vi "CRYSet ViewProperty XY  Front Panel.vi"(11 "Vi Ref":refnum<vi>) -> ()   [LabVIEW 2013]
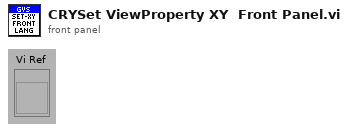
[diagram p1: front panel]
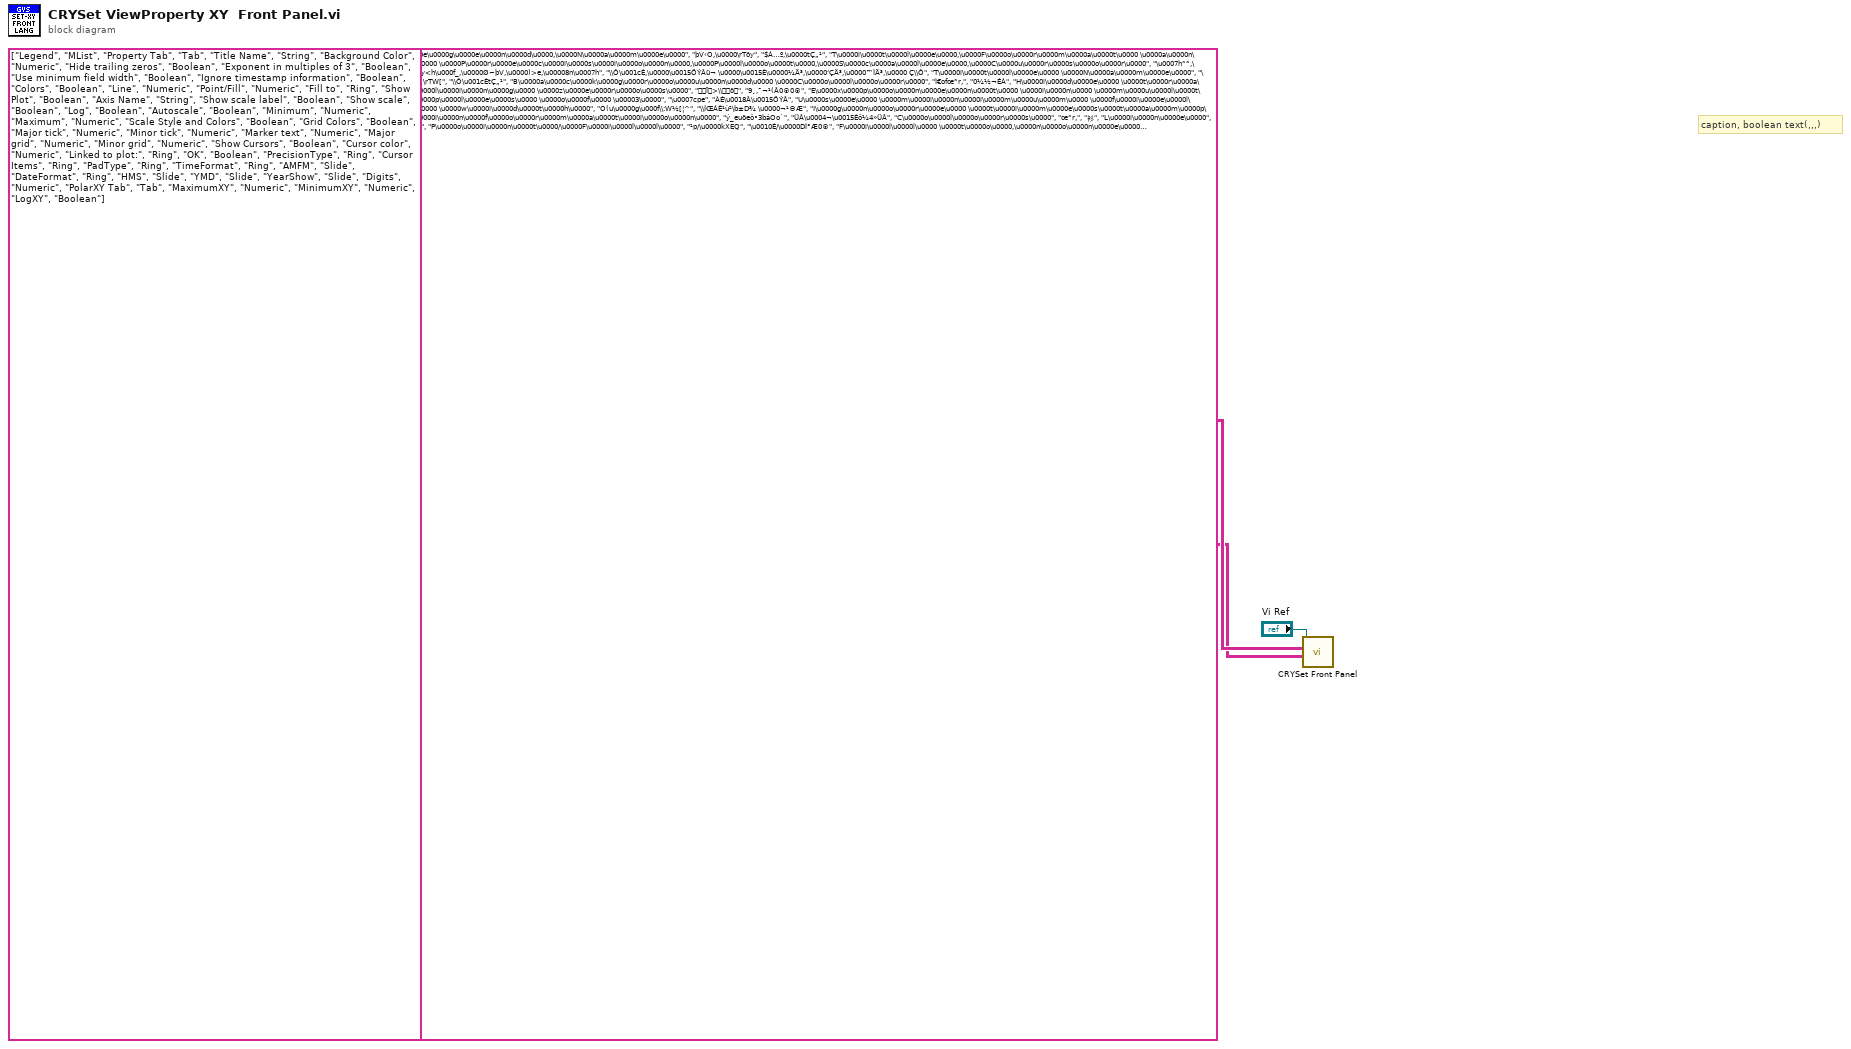
[diagram p0: block diagram]
diagram:
  # "Caption, Tab Page, Multilist Header, Button 4"
  # "Control Type"
  # "Control Name and Tab"
  # "caption, boolean text(,,,)"
  # "Caption/Boolean Text"
  n1 = call "CRYSet Front Panel.vi"("Caption(Boolean Text)"=string[][] [["L\u0000e\u0000g\u0000e\u0000n\u0000d\u0000,\u0000N\u0000a\u0000m\u0000e\u0000", "þV‹O,\u0000\rTðy", "$Á…º,\u0000tÇ„¹"], ["T\u0000i\u0000t\u0000l\u0000e\u0000,\u0000F\u0000o\u0000r\u0000m\u0000a\u0000t\u0000 \u0000a\u0000n\u0000d\u0000 \u0000P\u0000r\u0000e\u0000c\u0000i\u0000s\u0000i\u0000o\u0000n\u0000,\u0000P\u0000l\u0000o\u0000t\u0000,\u0000S\u0000c\u0000a\u0000l\u0000e\u0000,\u0000C\u0000u\u0000r\u0000s\u0000o\u0000r\u0000", "\u0007h˜˜,\u0000>f:y<h\u000f_,\u0000Ø~þV,\u0000)>e,\u00008n\u0007h", "\\Ô\u001cÈ,\u0000\u0015ÖÝÂü¬ \u0000\u0015È\u0000¼Ä³,\u0000‘ÇÄ³,\u0000™ÌÄ³,\u0000 Ç\\Ô"], ["T\u0000i\u0000t\u0000l\u0000e\u0000 \u0000N\u0000a\u0000m\u0000e\u0000", "\u0007h˜˜\rTW[", "\\Ô\u001cÈtÇ„¹"], ["B\u0000a\u0000c\u0000k\u0000g\u0000r\u0000o\u0000u\u0000n\u0000d\u0000 \u0000C\u0000o\u0000l\u0000o\u0000r\u0000", "Ì€ofœ˜r‚", "0¼½¬ÉÀ"], ["H\u0000i\u0000d\u0000e\u0000 \u0000t\u0000r\u0000a\u0000i\u0000l\u0000i\u0000n\u0000g\u0000 \u0000z\u0000e\u0000r\u0000o\u0000s\u0000", "Ï>\\ö", "9¸,¯¬¹(Â0®0®"], ["E\u0000x\u0000p\u0000o\u0000n\u0000e\u0000n\u0000t\u0000 \u0000i\u0000n\u0000 \u0000m\u0000u\u0000l\u0000t\u0000i\u0000p\u0000l\u0000e\u0000s\u0000 \u0000o\u0000f\u0000 \u00003\u0000", "\u0007cpe", "ÀÉ\u0018Â\u0015ÖÝÂ"], ["U\u0000s\u0000e\u0000 \u0000m\u0000i\u0000n\u0000i\u0000m\u0000u\u0000m\u0000 \u0000f\u0000i\u0000e\u0000l\u0000d\u0000 \u0000w\u0000i\u0000d\u0000t\u0000h\u0000", "O(u\u0000g\u000f\\:W½[¦^", "\\ÍŒÁÈ¹ù²\b±D¾ \u0000¬¹©Æ"], ["I\u0000g\u0000n\u0000o\u0000r\u0000e\u0000 \u0000t\u0000i\u0000m\u0000e\u0000s\u0000t\u0000a\u0000m\u0000p\u0000 \u0000i\u0000n\u0000f\u0000o\u0000r\u0000m\u0000a\u0000t\u0000i\u0000o\u0000n\u0000", "ý_euöeô•3báOo`", "ÜÂ\u0004¬\u0015Èô¼4»ÜÂ"], ["C\u0000o\u0000l\u0000o\u0000r\u0000s\u0000", "œ˜r‚", "衫"], ["L\u0000i\u0000n\u0000e\u0000", "¿~", " Á"], ["P\u0000o\u0000i\u0000n\u0000t\u0000/\u0000F\u0000i\u0000l\u0000l\u0000", "¹p/\u0000kXEQ", "\u0010È/\u0000DÌ°Æ0®"], ["F\u0000i\u0000l\u0000l\u0000 \u0000t\u0000o\u0000,\u0000n\u0000o\u0000n\u0000e\u0000,\u0000z\u0000e\u0000r\u0000o\u0000,\u0000-\u0000I\u0000n\u0000f\u0000i\u0000n\u0000i\u0000t\u0000y\u0000,\u0000+\u0000I\u0000n\u0000f\u0000i\u0000n\u0000i\u0000t\u0000y\u0000", "kX™Q,\u0000àe,\u0000ö–,\u0000-\u0000àewz,\u0000+\u0000àewz", "DÌ°Æ0®,\u0000n\u0000o\u0000n\u0000e\u0000,\u0000z\u0000e\u0000r\u0000o\u0000,\u0000-\u0000I\u0000n\u0000f\u0000i\u0000n\u0000i\u0000t\u0000y\u0000,\u0000+\u0000I\u0000n\u0000f\u0000i\u0000n\u0000i\u0000t\u0000y\u0000"], ["S\u0000h\u0000o\u0000w\u0000 \u0000P\u0000l\u0000o\u0000t\u0000", ">f:yØ~þV", "á¬ Áô¼ìÅüÈ0®"], ["N\u0000a\u0000m\u0000e\u0000", "\rTW[", "tÇ„¹"], ["S\u0000h\u0000o\u0000w\u0000 \u0000s\u0000c\u0000a\u0000l\u0000e\u0000 \u0000l\u0000a\u0000b\u0000e\u0000l\u0000", ">f:y)>e\u0007h~{", "™ÌÄ³tÇ„¹ô¼ìÅüÈ0®"], ["S\u0000h\u0000o\u0000w\u0000 \u0000s\u0000c\u0000a\u0000l\u0000e\u0000", ">f:y)>e", "™ÌÄ³ô¼ìÅüÈ0®"], ["L\u0000o\u0000g\u0000", "ù[pe", "\\¸ø­"], ["A\u0000u\u0000t\u0000o\u0000s\u0000c\u0000a\u0000l\u0000e\u0000", "ꁨR)>e", "ÇÙ³ÌÄ³"], ["M\u0000i\u0000n\u0000i\u0000m\u0000u\u0000m\u0000", "\u0000g\u000f\\<P", "\\ÍŒÁ\u0012¬"], ["M\u0000a\u0000x\u0000i\u0000m\u0000u\u0000m\u0000", "\u0000g'Y<P", "\\Í\u0000³\u0012¬"], ["S\u0000c\u0000a\u0000l\u0000e\u0000 \u0000S\u0000t\u0000y\u0000l\u0000e\u0000 \u0000a\u0000n\u0000d\u0000 \u0000C\u0000o\u0000l\u0000o\u0000r\u0000s\u0000", ")>e7h\u000f_ŒTœ˜r‚", "™ÌÄ³\u0015ÖÝÂü¬ \u0000ÉÀ"], ["G\u0000r\u0000i\u0000d\u0000 \u0000C\u0000o\u0000l\u0000o\u0000r\u0000s\u0000", "Q<hœ˜r‚", "©¬ÇÉÀ\b¬"], ["M\u0000a\u0000j\u0000o\u0000r\u0000 \u0000t\u0000i\u0000c\u0000k\u0000", ";N;R¦^", "0®ø¼\b²\b®"], ["M\u0000i\u0000n\u0000o\u0000r\u0000 \u0000t\u0000i\u0000c\u0000k\u0000", ";R¦^", "ô¼pÈ\b²\b®"], ["M\u0000a\u0000r\u0000k\u0000e\u0000r\u0000 \u0000t\u0000e\u0000x\u0000t\u0000", "\u0007h°‹‡e,g", "ÌÄ³\\ÔÝÂ8»Ç"], ["M\u0000a\u0000j\u0000o\u0000r\u0000 \u0000g\u0000r\u0000i\u0000d\u0000", ";NQ<h", "0®ø¼©¬Ç"], ["M\u0000i\u0000n\u0000o\u0000r\u0000 \u0000g\u0000r\u0000i\u0000d\u0000", "Q<h", "ô¼pÈ©¬Ç"], ["S\u0000h\u0000o\u0000w\u0000 \u0000C\u0000u\u0000r\u0000s\u0000o\u0000r\u0000s\u0000", ">f:y8n\u0007h", " Ç\\Ôô¼ìÅüÈ0®"], ["C\u0000u\u0000r\u0000s\u0000o\u0000r\u0000 \u0000c\u0000o\u0000l\u0000o\u0000r\u0000", "8n\u0007hœ˜r‚", " Ç\\ÔÉÀ"], ["L\u0000i\u0000n\u0000k\u0000e\u0000d\u0000 \u0000t\u0000o\u0000 \u0000p\u0000l\u0000o\u0000t\u0000:\u0000", "Þ¥c0R8n\u0007h", " Ç\\Ô(¸°¬"], ["O\u0000K\u0000", "nx¤‹", "UÖxÇ"], ["P\u0000r\u0000e\u0000c\u0000i\u0000s\u0000i\u0000o\u0000n\u0000T\u0000y\u0000p\u0000e\u0000,\u0000D\u0000i\u0000g\u0000i\u0000t\u0000a\u0000l\u0000s\u0000 \u0000o\u0000f\u0000 \u0000p\u0000r\u0000e\u0000c\u0000i\u0000s\u0000i\u0000o\u0000n\u0000,\u0000S\u0000i\u0000g\u0000n\u0000i\u0000f\u0000i\u0000c\u0000a\u0000n\u0000t\u0000 \u0000d\u0000i\u0000g\u0000i\u0000t\u0000s\u0000", "¾|¦^{|‹W,\u0000¾|¦^MOpe,\u0000\tgHepeW[", "\u0015È\u0000¼Ä³\u0015ÖÝÂ,\u0000D\u0000i\u0000g\u0000i\u0000t\u0000a\u0000l\u0000s\u0000 \u0000o\u0000f\u0000 \u0000p\u0000r\u0000e\u0000c\u0000i\u0000s\u0000i\u0000o\u0000n\u0000,\u0000S\u0000i\u0000g\u0000n\u0000i\u0000f\u0000i\u0000c\u0000a\u0000n\u0000t\u0000 \u0000d\u0000i\u0000g\u0000i\u0000t\u0000s\u0000"], ["C\u0000u\u0000r\u0000s\u0000o\u0000r\u0000 \u0000I\u0000t\u0000e\u0000m\u0000s\u0000", "8n\u0007hy˜îv", " Ç\\ÔmÕ©º"], ["P\u0000a\u0000d\u0000T\u0000y\u0000p\u0000e\u0000,\u0000P\u0000a\u0000d\u0000 \u0000w\u0000i\u0000t\u0000h\u0000 \u0000s\u0000p\u0000a\u0000c\u0000e\u0000s\u0000 \u0000o\u0000n\u0000 \u0000l\u0000e\u0000f\u0000t\u0000,\u0000P\u0000a\u0000d\u0000 \u0000w\u0000i\u0000t\u0000h\u0000 \u0000s\u0000p\u0000a\u0000c\u0000e\u0000s\u0000 \u0000o\u0000n\u0000 \u0000r\u0000i\u0000g\u0000h\u0000t\u0000,\u0000P\u0000a\u0000d\u0000 \u0000w\u0000i\u0000t\u0000h\u0000 \u0000z\u0000e\u0000r\u0000o\u0000s\u0000 \u0000o\u0000n\u0000 \u0000l\u0000e\u0000f\u0000t\u0000", "kXEQ{|‹W,\u0000(Wæ] Rzz<h,\u0000(WóS Rzz<h,\u0000(Wæ] Rö–", "DÌÀÆ\u0015ÖÝÂ,\u0000|Æ½ÊÐÅ \u0000õ¬1¼DÌ°Æ0®,\u0000$Æx¹½ÊÐÅ \u0000õ¬1¼DÌ°Æ0®,\u0000|Æ½ÊÐÅ \u00009¸DÌ°Æ0®"], ["T\u0000i\u0000m\u0000e\u0000 \u0000F\u0000o\u0000r\u0000m\u0000a\u0000t\u0000", "öeô•<h\u000f_", "ÜÂ\u0004¬\u0015ÖÝÂ"], ["A\u0000M\u0000F\u0000M\u0000,\u0000A\u0000u\u0000t\u0000o\u0000,\u0000M\u0000a\u0000n\u0000u\u0000a\u0000l\u0000", "A\u0000M\u0000F\u0000M\u0000,\u0000ê¨R,\u0000Kb¨R", "$Æ\u0004È$ÆÄÖ,\u0000ÇÙ³,\u0000\u0018ÂÙ³"], ["D\u0000a\u0000t\u0000e\u0000 \u0000F\u0000o\u0000r\u0000m\u0000a\u0000t\u0000", "åe\u001fg<h\u000f_", " °Ç\u0015ÖÝÂ"], ["H\u0000M\u0000S\u0000,\u0000H\u0000H\u0000:\u0000M\u0000M\u0000,\u0000H\u0000H\u0000:\u0000M\u0000M\u0000:\u0000S\u0000S\u0000", "H\u0000M\u0000S\u0000,\u0000öe:\u0000\u0006R,\u0000öe:\u0000\u0006R:\u0000Òy", "ÜÂ„½\bÍ,\u0000ÜÂ:\u0000„½,\u0000ÜÂ:\u0000„½:\u0000\bÍ"], ["Y\u0000M\u0000D\u0000,\u0000M\u0000/\u0000D\u0000/\u0000Y\u0000,\u0000D\u0000/\u0000M\u0000/\u0000Y\u0000,\u0000Y\u0000/\u0000M\u0000/\u0000D\u0000", "\bgået^,\u0000\bg/\u0000åe/\u0000t^,\u0000åe/\u0000\bg/\u0000t^,\u0000t^/\u0000\bg/\u0000åe", "D±ÔÆ|Ç,\u0000ÔÆ/\u0000|Ç/\u0000D±,\u0000|Ç/\u0000ÔÆ/\u0000D±,\u0000D±/\u0000ÔÆ/\u0000|Ç"], ["Y\u0000e\u0000a\u0000r\u0000S\u0000h\u0000o\u0000w\u0000,\u0000D\u0000o\u0000 \u0000n\u0000o\u0000t\u0000 \u0000s\u0000h\u0000o\u0000w\u0000 \u0000y\u0000e\u0000a\u0000r\u0000,\u00002\u0000-\u0000d\u0000i\u0000g\u0000i\u0000t\u0000 \u0000y\u0000e\u0000a\u0000r\u0000,\u00004\u0000-\u0000d\u0000i\u0000g\u0000i\u0000t\u0000 \u0000y\u0000e\u0000a\u0000r\u0000", "t^>f:y,\u0000t^\rN>f:y,\u00002\u0000-\u0000MOP[,\u00004\u0000-\u0000MOP[", "D±Ä³ô¼ìÅüÈ0®,\u0000ô¼ìÅüÈÀÉJÅLÇ,\u00002\u0000Ç¬¹\u0018Â,\u00004\u0000Ç¬¹\u0018Â"], ["D\u0000i\u0000g\u0000i\u0000t\u0000s\u0000", "peW[", "\u0018ÂÇ"], ["F\u0000o\u0000r\u0000m\u0000a\u0000t\u0000 \u0000a\u0000n\u0000d\u0000 \u0000P\u0000r\u0000e\u0000c\u0000i\u0000s\u0000i\u0000o\u0000n\u0000,\u0000P\u0000l\u0000o\u0000t\u0000,\u0000S\u0000c\u0000a\u0000l\u0000e\u0000", ">f:y<h\u000f_,\u0000Ø~þV,\u0000)>e", "\u0015ÖÝÂü¬ \u0000\u0015È\u0000¼Ä³,\u0000‘ÇÄ³,\u0000™ÌÄ³"], ["M\u0000a\u0000x\u0000i\u0000m\u0000u\u0000m\u0000", "\u0000g'Y<P", "\\Í\u0000³\u0012¬"], ["M\u0000i\u0000n\u0000i\u0000m\u0000u\u0000m\u0000", "\u0000g\u000f\\<P", "\\ÍŒÁ\u0012¬"], ["L\u0000o\u0000g\u0000", "ù[pe", "\\¸ø­"]], "Control ID and Type(Label Name, Type)"=string[][] [["Legend", "MList"], ["Property Tab", "Tab"], ["Title Name", "String"], ["Background Color", "Numeric"], ["Hide trailing zeros", "Boolean"], ["Exponent in multiples of 3", "Boolean"], ["Use minimum field width", "Boolean"], ["Ignore timestamp information", "Boolean"], ["Colors", "Boolean"], ["Line", "Numeric"], ["Point/Fill", "Numeric"], ["Fill to", "Ring"], ["Show Plot", "Boolean"], ["Axis Name", "String"], ["Show scale label", "Boolean"], ["Show scale", "Boolean"], ["Log", "Boolean"], ["Autoscale", "Boolean"], ["Minimum", "Numeric"], ["Maximum", "Numeric"], ["Scale Style and Colors", "Boolean"], ["Grid Colors", "Boolean"], ["Major tick", "Numeric"], ["Minor tick", "Numeric"], ["Marker text", "Numeric"], ["Major grid", "Numeric"], ["Minor grid", "Numeric"], ["Show Cursors", "Boolean"], ["Cursor color", "Numeric"], ["Linked to plot:", "Ring"], ["OK", "Boolean"], ["PrecisionType", "Ring"], ["Cursor Items", "Ring"], ["PadType", "Ring"], ["TimeFormat", "Ring"], ["AMFM", "Slide"], ["DateFormat", "Ring"], ["HMS", "Slide"], ["YMD", "Slide"], ["YearShow", "Slide"], ["Digits", "Numeric"], ["PolarXY Tab", "Tab"], ["MaximumXY", "Numeric"], ["MinimumXY", "Numeric"], ["LogXY", "Boolean"]], "Vi Ref"="Vi Ref") -> ()  [unwired: 9 in]
